vi "Pos_Calculate Frame Starting Position.vi"(4 "Width":u32, 5 "Max Width":u32=32, 6 "Height":u32, 7 "Max Height":u32=32, 8 "Error":errorcluster, 11 "Position":T2) -> (0 "Error Out":errorcluster, 3 "Postion Out":T1)   [LabVIEW 2025]
uses:
  TypeDefs_Utility/ENUM RB_Pos_Quadrant Position.ctl
  TypeDefs_Utility/Cluster_Top Left position.ctl
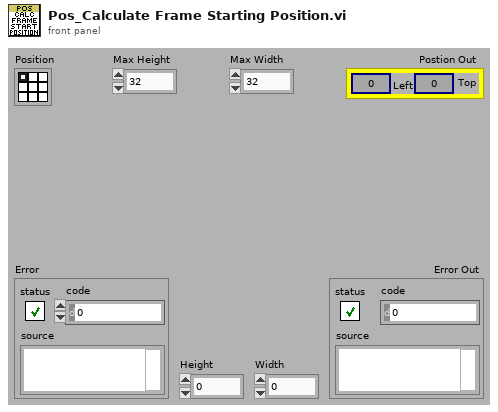
[diagram p1: front panel]
types:
  T1 = typedef "Cluster_Top Left position.ctl" = cluster{"Left":i32, "Top":i32}
  T2 = typedef "ENUM RB_Pos_Quadrant Position.ctl" = enum32{"LFT-TOP", "MID-TOP", "RGT-TOP", "LFT-CTR", "MID-CTR", "RGT-CTR", "LFT-BOT", "MID-BOT", "RGT-BOT"}
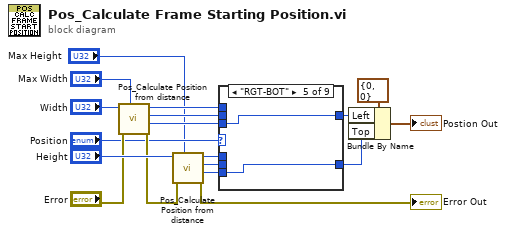
[diagram p0: block diagram]
diagram:
  n1 = call "Pos_Calculate Position from distance.vi"("Space size"="Max Width", "Error"="Error", "Distance"="Width") -> ("Error Out"=w13:errorcluster, "Far Position Out"=w6:i32, "Center Position Out"=w9:i32, "Near Positoin Out"=w5:i32)  [unwired: 5 in]
  n2 = call "Pos_Calculate Position from distance.vi"("Space size"="Max Height", "Error"=w13, "Distance"="Height") -> ("Error Out"=→"Error Out":errorcluster, "Far Position Out"=w4:i32, "Center Position Out"=w8:i32, "Near Positoin Out"=w3:i32)  [unwired: 5 in]
  n3 = case shown="\"RGT-BOT\"" "Position" {
    tunnel: w9 -> [w20 _ _ w25 _ w29 _ _ _]
    tunnel: [w20 w21 w23 w25 w27 w29 w31 w33 w36] -> w10
    tunnel: [w19 w22 w24 w26 w28 w30 w32 w34 w35] -> w7
    tunnel: w8 -> [w19 w22 _ _ _ _ _ w34 _]
    tunnel: w6 -> [_ w21 _ _ w27 _ w31 _ _]
    tunnel: w5 -> [_ _ w23 _ _ _ _ w33 w36]
    tunnel: w4 -> [_ _ w24 w26 w28 _ _ _ _]
    tunnel: w3 -> [_ _ _ _ _ w30 w32 _ w35]
    frame "MID-CTR" {
    }
    frame "RGT-CTR" {
    }
    frame "LFT-BOT" {
    }
    frame "MID-BOT" {
    }
    frame "RGT-BOT" {
    }
    frame "MID-TOP" {
    }
    frame "RGT-TOP" {
    }
    frame "LFT-CTR" {
    }
    frame "LFT-TOP" {
    }
  }
  n4 = Bundle By Name(cluster=T1 {"Left"=0, "Top"=0} ("Postion"), "Left"=w10, "Top"=w7) -> (→"Postion Out":T1)
